vi "Trace Results.vi"(9 "Status of previous command":T3, 10 "Description":string, 11 "Subsystem":string) -> ()   [LabVIEW 2017]
doc: "This VI displays the execution trace of various commands and subsystems. Use command descriptions and controller print formatting to make it easier to understand the trace."
uses:
  <vilib>/Rock Robotics/WPI/Framework/Completion Status.ctl
panel:
  in  "Number of Traces":i32=200
  in  "Tab Control":T1(tab)
  out "Subsystem Trace":T2(array[cluster])
  out "Details":string
  out "XY Graph":cluster{"Tracings":cluster{dbl, dbl}[]}[](graph)
  in  "Clear":bool
  in  "Show Default Cmds":bool
  in  "Trace Enable":bool
  # "Default"
  # "Aborted"
  # "Successful"
  # "Ongoing"
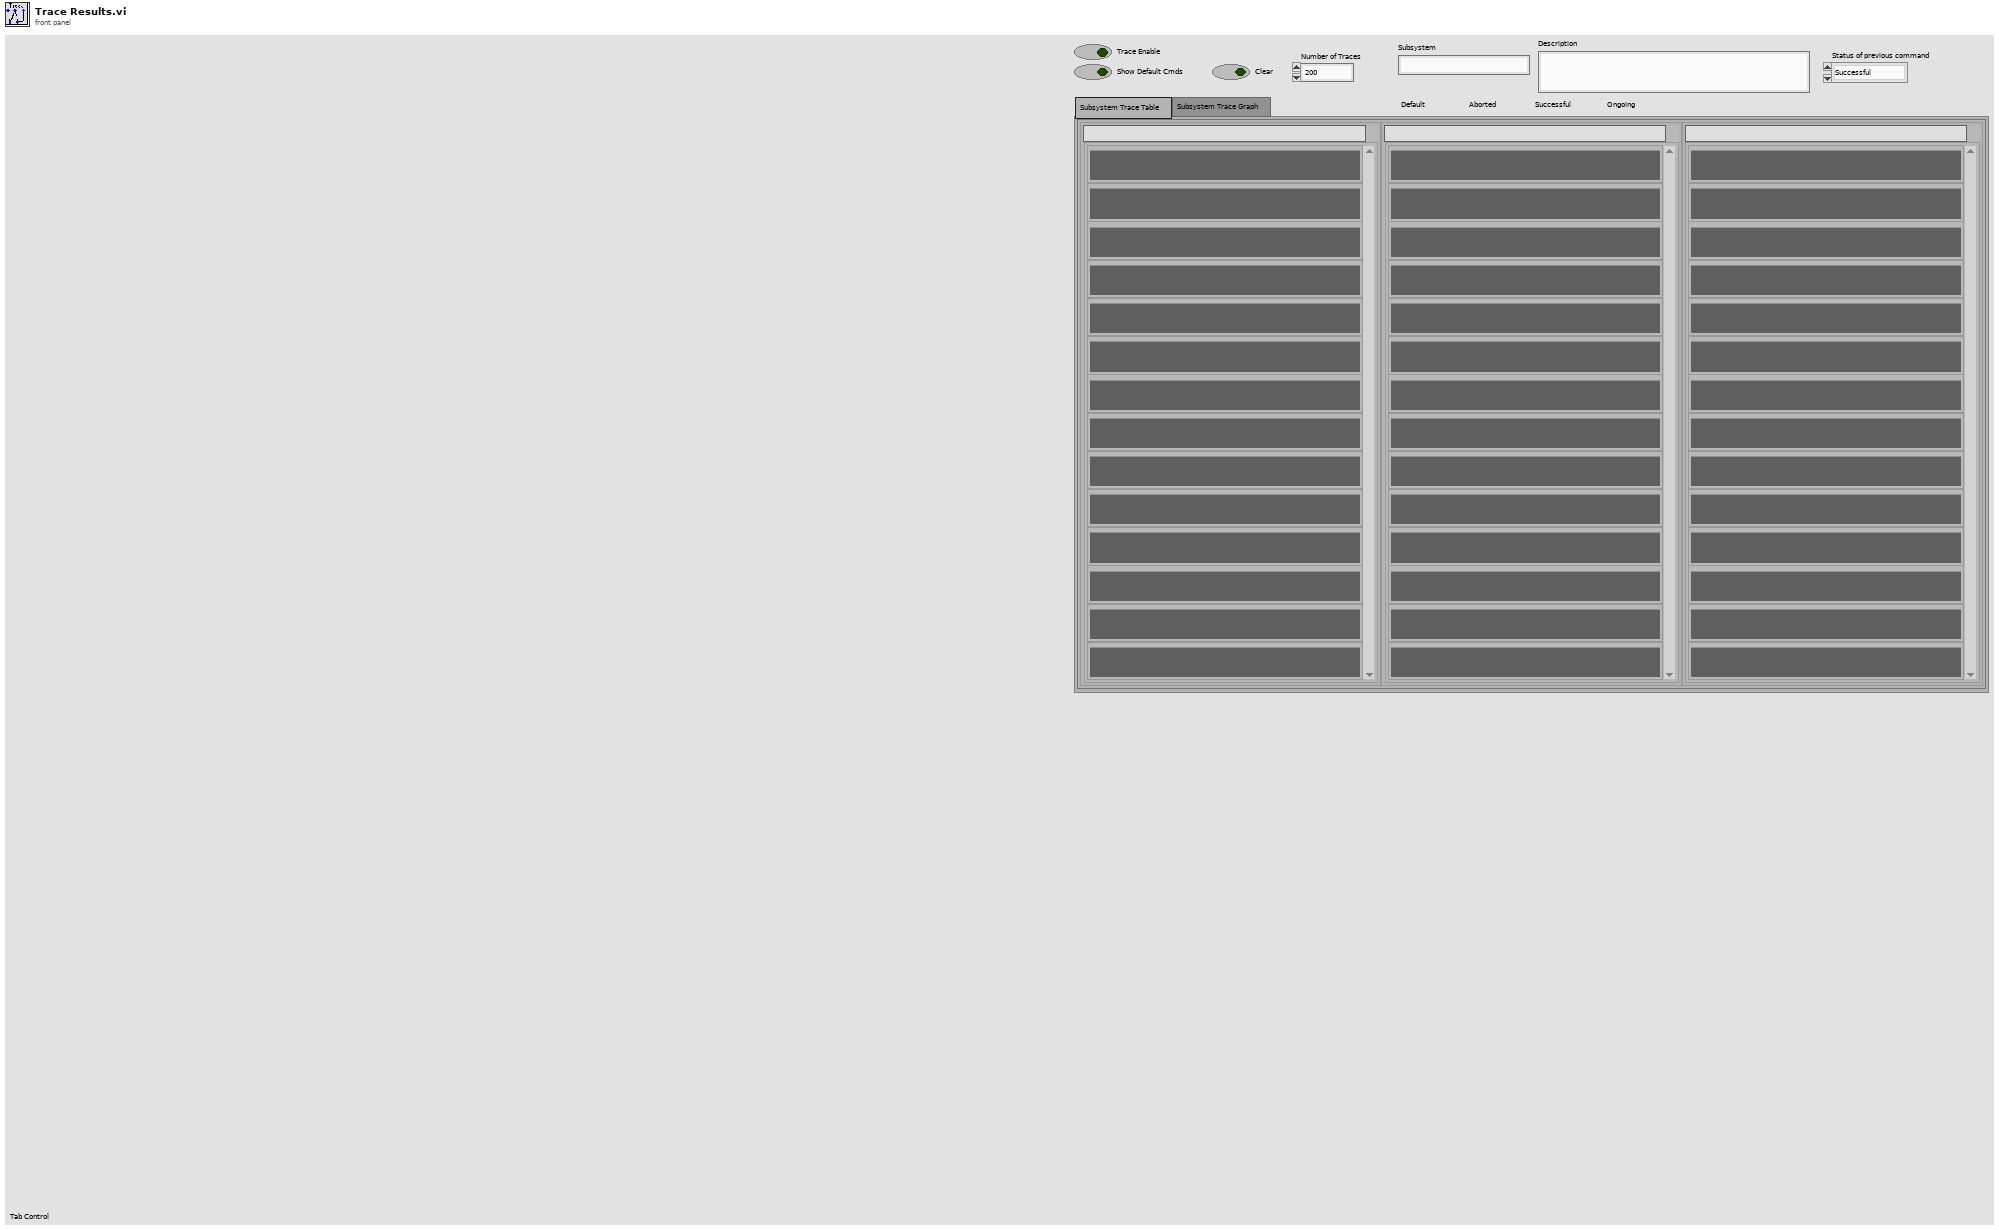
[diagram p1: front panel]
types:
  T1 = enum32{"Subsystem Trace Table", "Subsystem Trace Graph"}
  T2 = cluster{"Subsystem":string, "Tracings":cluster{"Command":string, "Color":u32}[]}[]
  T3 = typedef "Completion Status.ctl" = enum16{"Successful", "Aborted", "Incomplete"}
  T4 = cluster{"Subsystem":string, "Tracings":cluster{"Command":string, "Color":u32}[]}
  T5 = cluster{"Subsystem":string, cluster{"Description":string, "Active":u32}[]}
  T6 = cluster{"Subsystem":string, "Tracings":cluster{"Description":string, "Active":u32}[]}[]
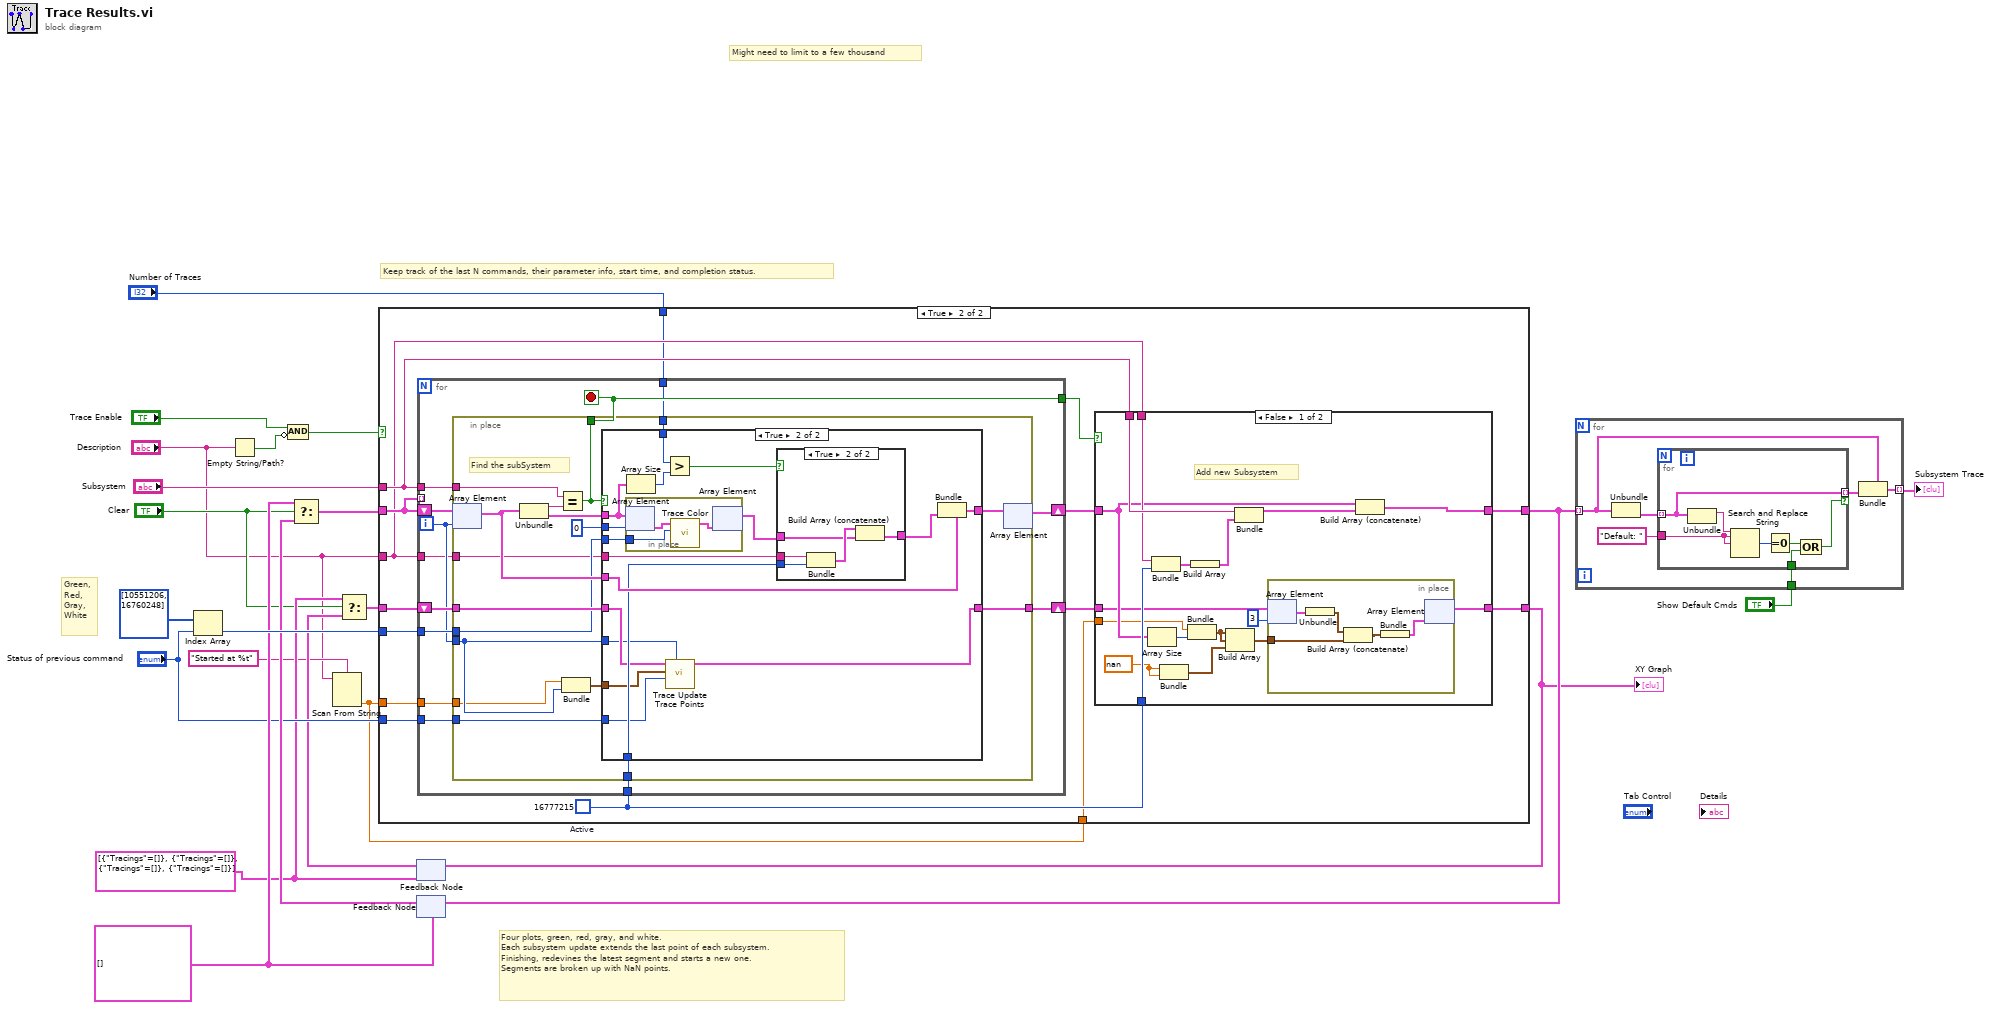
[diagram p0: block diagram]
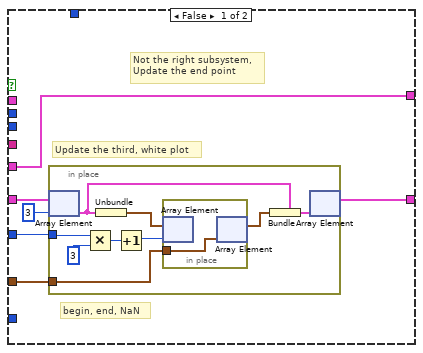
[diagram p4: hidden frame]
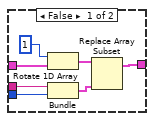
[diagram p5: hidden frame]
diagram:
  w5 = cluster{"Tracings":cluster{dbl, dbl}[]}[] [{"Tracings"=[]}, {"Tracings"=[]}, {"Tracings"=[]}, {"Tracings"=[]}]
  w10 = T2 []
  # "Green,\nRed,\nGray,\nWhite"
  # "Four plots, green, red, gray, and white.\nEach subsystem update extends the last point of each subsystem.\nFinishing, redevines the latest segment and starts a new one.\nSegments are broken up with NaN points."
  # "Keep track of the last N commands, their parameter info, start time, and completion status."
  # "Might need to limit to a few thousand"
  n1 = Index Array(array=u32[] [10551206, 16760248], index="Status of previous command") -> (element=w18:u32)
  n2 = Empty String/Path?(string/path="Description") -> (empty?=w22:bool)
  n3 = Compound Arithmetic op=AND("Trace Enable", invert w22) -> (w19:bool)
  n4 = Scan From String(format string="Started at %t", input string="Description") -> (output 1=w1:dbl)  [unwired: 3 in, 3 out]
  n5 = feedback #1(w5) -> (w6:cluster{"Tracings":cluster{dbl, dbl}[]}[])
  n6 = Select(t=w5, s="Clear", f=w6) -> (s? t:f=w7:cluster{"Tracings":cluster{dbl, dbl}[]}[])
  n7 = feedback #2(w10) -> (w13:T2)
  n8 = Select(t=w10, s="Clear", f=w13) -> (s? t:f=w12:T2)
  n9 = case shown="True" w19 {
    tunnel: w12 -> [w24 w39]
    tunnel: "Subsystem" -> [_ w36]
    tunnel: "Description" -> [_ w35]
    tunnel: [w24 w34] -> w16
    tunnel: w18 -> [_ w33]
    tunnel: "Number of Traces" -> [_ w32]
    tunnel: w7 -> [w23 w31]
    tunnel: [w23 w29] -> w8
    tunnel: "Status of previous command" -> [_ w27]
    tunnel: w1 -> [_ w26]
    tunnel: w1 -> [_ w25]
    frame False {
    }
    frame True {
      w28 = u32 16777215  # Active
      n10 = for {
        tunnel: w36 -> [w76]
        tunnel: w35 -> [w65]
        shift-right: [w74] -> w37
        shift-left: w39 -> [w75]
        tunnel: [w73] -> w38
        tunnel: w39 -> [_] mode=indexing
        tunnel: w28 -> [w72]
        tunnel: w33 -> [w71]
        tunnel: w32 -> [w70]
        shift-right: [w67] -> w30
        shift-left: w31 -> [w69]
        tunnel: w27 -> [w66]
        tunnel: w26 -> [w64]
        i -> [w68]
        stop <- w73 stop-if-true
        n11 = in-place {
          in-place-border: w76 -> [w92]
          in-place-border: w65 -> [w78]
          in-place-border: [w88] -> w73
          in-place-border: w72 -> [w87]
          in-place-border: w71 -> [w80]
          in-place-border: w70 -> [w85]
          in-place-border: w69 -> [w84]
          in-place-border: w68 -> [w83]
          in-place-border: [w81] -> w67
          in-place-border: w66 -> [w79]
          in-place-border: w64 -> [w77]
          # "Find the subSystem"
          n12 = in-place-array #3(w75, w68) -> (w89:T4)
          n13 = Unbundle(w89) -> ("Subsystem"=w93:string, "Tracings"=w91:cluster{"Command":string, "Color":u32}[])
          n14 = Equal?(x=w92, y=w93) -> (x = y?=w88:bool)
          n15 = Bundle(w77, w83) -> (w82:cluster{dbl, i32})  [unwired: 1 in]
          n16 = case shown="True" w88 {
            tunnel: w91 -> [_ w122]
            tunnel: w78 -> [_ w126]
            tunnel: [w99 w125] -> w90
            tunnel: w89 -> [w99 w124]
            tunnel: w87 -> [_ w116]
            tunnel: 0 -> [_ w120]
            tunnel: w85 -> [_ w119]
            tunnel: w84 -> [w98 w113]
            tunnel: w83 -> [w96 w110]
            tunnel: w82 -> [w95 w114]
            tunnel: [w94 w112] -> w81
            tunnel: w80 -> [_ w115]
            tunnel: w79 -> [_ w111]
            frame False {
              # "Update the third, white plot"
              # "Not the right subsystem,\nUpdate the end point"
              # "begin, end, NaN"
              n17 = in-place {
                in-place-border: w96 -> [w107]
                in-place-border: w95 -> [w103]
                n18 = in-place-array #4(w98, 3) -> (w106:cluster{"Tracings":cluster{dbl, dbl}[]})
                n19 = Multiply(x=w107, y=3) -> (x*y=w101:i32)
                n20 = Unbundle(w106) -> ("Tracings"=w102:cluster{dbl, dbl}[])
                n21 = Increment(x=w101) -> (x+1=w100:i32)
                n22 = in-place {
                  in-place-border: w103 -> [w109]
                  n23 = in-place-array #5(w102, w100) -> ()  [unwired: 1 out]
                  n24 = in-place-array #5(w109) -> (w104:cluster{dbl, dbl}[])  [unwired: 1 out]
                }
                n25 = Bundle(cluster=w106, "Tracings"=w104) -> (w105:cluster{"Tracings":cluster{dbl, dbl}[]})
                n26 = in-place-array #4(w105) -> (w94:cluster{"Tracings":cluster{dbl, dbl}[]}[])  [unwired: 1 out]
              }
            }
            frame True {
              n27 = in-place {
                in-place-border: w115 -> [w139]
                n28 = in-place-array #6(w122, w120) -> (w141:cluster{"Command":string, "Color":u32})
                n29 = call <vilib>:"Trace Color.vi"("Color"=w139, "Cluster in"=w141) -> ("Cluster out"=w140:cluster{"Command":string, "Color":u32})  [unwired: 9 in]
                n30 = in-place-array #6(w140) -> (w121:cluster{"Command":string, "Color":u32}[])  [unwired: 1 out]
              }
              n31 = Array Size(array=w122) -> (size(s)=w118:i32)
              n32 = Greater?(x=w119, y=w118) -> (0:w117:bool)
              n33 = call <vilib>:"Trace Update Trace Points.vi"("index"=w110, "Status of previous command"=w111, "New Point"=w114, "Array in"=w113) -> ("Array out"=w112:cluster{"Tracings":cluster{dbl, dbl}[]}[])  [unwired: 7 in]
              n34 = case shown="True" w117 {
                tunnel: w121 -> [w133 w134]
                tunnel: w126 -> [w130 w137]
                tunnel: [w129 w138] -> w123
                tunnel: w116 -> [w127 w135]
                frame False {
                  n35 = Rotate 1D Array(1:w133, 2:1 ("n")) -> (0:w131:cluster{"Command":string, "Color":u32}[])
                  n36 = Bundle("Description"=w130, "Active"=w127) -> (w128:cluster{"Description":string, "Active":u32})  [unwired: 1 in]
                  n37 = Replace Array Subset(array=w131, new element=w128) -> (w129:cluster{"Command":string, "Color":u32}[])  [unwired: 1 in]
                }
                frame True {
                  n38 = Bundle("Description"=w137, "Active"=w135) -> (w136:cluster{"Description":string, "Active":u32})  [unwired: 1 in]
                  n39 = Build Array (concatenate)(w136, w134) -> (w138:cluster{"Command":string, "Color":u32}[])
                }
              }
              n40 = Bundle(cluster=w124, "Tracings"=w123) -> (w125:T4)  [unwired: 1 in]
            }
          }
          n41 = in-place-array #3(w90) -> (w74:T2)  [unwired: 1 out]
        }
      }
      n42 = case shown="False" w38 {
        tunnel: w37 -> [w49 w63]
        tunnel: [w51 w63] -> w34
        tunnel: w36 -> [w55 _]
        tunnel: w35 -> [w53 _]
        tunnel: w28 -> [w50 _]
        tunnel: w30 -> [w42 w62]
        tunnel: [w40 w62] -> w29
        tunnel: w25 -> [w47 _]
        frame False {
          w45 = nan
          # "Add new Subsystem"
          n43 = Array Size(array=w49) -> (size(s)=w48:i32)
          n44 = Bundle("Description"=w53, "Active"=w50) -> (w56:cluster{"Description":string, "Active":u32})  [unwired: 1 in]
          n45 = Bundle(w45, w45) -> (w44:cluster{dbl, dbl})  [unwired: 1 in]
          n46 = Bundle(w47, w48) -> (w43:cluster{dbl, i32})  [unwired: 1 in]
          n47 = Build Array(w56) -> (w54:cluster{"Description":string, "Active":u32}[])
          n48 = Build Array(w43, w43, w44) -> (w46:cluster{dbl, dbl}[])
          n49 = Bundle("Subsystem"=w55, w54) -> (w52:T5)  [unwired: 1 in]
          n50 = in-place {
            in-place-border: w46 -> [w59]
            n51 = in-place-array #7(w42, 3) -> (w61:cluster{"Tracings":cluster{dbl, dbl}[]})
            n52 = Unbundle(w61) -> ("Tracings"=w60:cluster{dbl, dbl}[])
            n53 = Build Array (concatenate)(w60, w59) -> (w58:cluster{dbl, dbl}[])
            n54 = Bundle(w58) -> (w57:cluster{cluster{dbl, dbl}[]})  [unwired: 1 in]
            n55 = in-place-array #7(w57) -> (w40:cluster{"Tracings":cluster{dbl, dbl}[]}[])  [unwired: 1 out]
          }
          n56 = Build Array (concatenate)(w49, w52) -> (w51:T6)
        }
        frame True {
        }
      }
    }
  }
  "XY Graph" <- w8
  n57 = feedback-in #1(w8) -> ()
  n58 = feedback-in #2(w16) -> ()
  n59 = for {
    tunnel: w16 -> [w144] mode=indexing
    tunnel: "Show Default Cmds" -> [w146]
    tunnel: [w142] -> w14 mode=indexing
    n60 = Unbundle(w144) -> ("Tracings"=w145:cluster{"Command":string, "Color":u32}[])  [unwired: 1 out]
    n61 = for {
      tunnel: "Default: " -> [w152]
      tunnel: w146 -> [w151]
      tunnel: w145 -> [w149] mode=indexing
      tunnel: [w149] -> w143 mode=indexing if=w150
      n62 = Unbundle(w149) -> ("Command"=w148:string)  [unwired: 1 out]
      n63 = Search and Replace String(input string=w148, search string=w152, replace string=w152) -> (number of replacements=w153:i32)  [unwired: 5 in, 3 out]
      n64 = Equal To 0?(x=w153) -> (x = 0?=w154:bool)
      n65 = Compound Arithmetic op=OR(w154, w151) -> (w150:bool)
    }
    n66 = Bundle(cluster=w144, "Tracings"=w143) -> (w142:T4)  [unwired: 1 in]
  }
  "Subsystem Trace" <- w14
